vi "Add Database.vi"(7 "Highlight? (F)":bool, 8 "error in":errorcluster, 9 "Path":path, 10 "Name":string, 11 "Parent Ref":T1 format="%.0x") -> (0 "error out":errorcluster)   [LabVIEW 2020, in "Communication Bus Template Scripting.lvlib"]
uses:
  <vilib>/NI VeriStand/Custom Device API/Custom Device Item Ref.ctl
  Shared/Constants.vi
  <vilib>/NI VeriStand/Custom Device API/Set Item Property (Path).vi
  Communication Bus Template Scripting.lvlib
  <vilib>/NI VeriStand/Custom Device API/Custom Device API.lvlib
  Shared/Communication Bus Template Shared.lvlib
panel:
  out "Database Ref out":T1 format="%.0x"
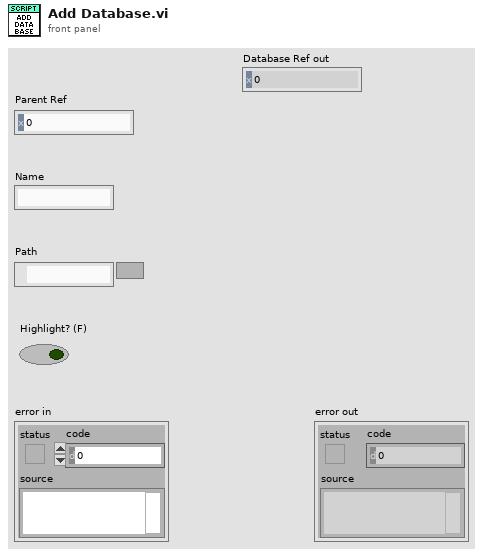
[diagram p1: front panel]
types:
  T1 = typedef "Custom Device API.lvlib/Custom Device Item Ref.ctl" = u64
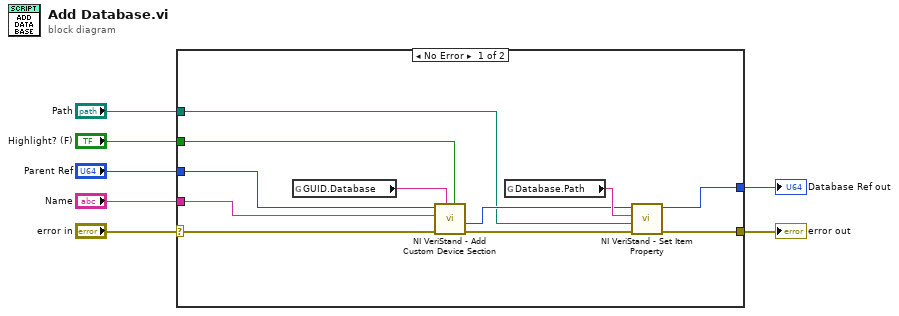
[diagram p0: block diagram]
diagram:
  n1 = case shown="No Error" "error in" {
    selector: "error in" -> [w9 w19]
    tunnel: "Name" -> [w15 _]
    tunnel: "Parent Ref" -> [w14 _]
    tunnel: [w12 w19] -> w5
    tunnel: "Path" -> [w11 _]
    tunnel: "Highlight? (F)" -> [w10 _]
    tunnel: [w8 _] -> w1
    frame No Error {
      n2 = global read "Constants.vi" "GUID.Database"() -> (w13:string)
      n3 = call <vilib>:"NI VeriStand - Add Custom Device Section.vi"("Highlight? (F)"=w10, "GUID (Default Section)"=w13, "error in (no error)"=w9, "Section Name"=w15, "Parent Ref in"=w14) -> ("error out"=w16:errorcluster, "Section Ptr"=w17:T1)  [unwired: 3 in, 2 out]
      n4 = global read "Constants.vi" "Database.Path"() -> (w18:string)
      n5 = call-poly <vilib>:"NI VeriStand - Set Item Property.vi"("error in (no error)"=w16, "Value"=w11, "Property Name"=w18, "Item Ref in"=w17) -> ("error out"=w12:errorcluster, "Item Ref out"=w8:T1)  [unwired: 5 in, 1 out]
    }
    frame Error {
    }
  }
  "error out" <- w5
  "Database Ref out" <- w1
